vi "Generate Data.vi"() -> ()   [LabVIEW 2010]
doc: "이 VI는 LabVIEW Core II의 글로벌 데이터 프로젝트 연습문제에 대한 해답입니다.\n\n이 프로젝트를 실행하려면, 글로벌 데이터(Global Data) LV 프로젝트 파일을 열고, 데이터 생성(Generate Data) VI와 데이터 읽기(Read Data) VI를 열고, 실행하십시오. 데이터는 데이터 생성 VI에서 생성되며 데이터 읽기 VI에서 표시됩니다. 데이터 생성 VI와 데이터 읽기 VI는 하나의 정지 버튼을 공유합니다."
panel:
  out "데이터":dbl
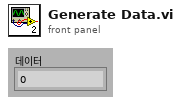
[diagram p1: front panel]
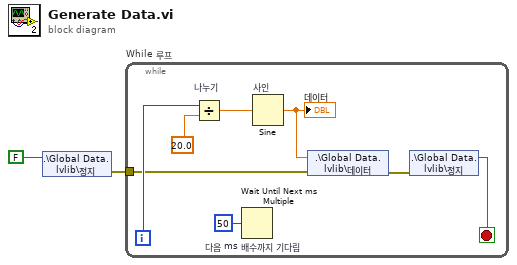
[diagram p0: block diagram]
diagram:
  n1 = shared-variable ".\\Global Data.lvlib\\정지"(FALSE ("Stop")) -> (error out=w1:errorcluster)  [unwired: 1 in]
  n2 = while "While 루프" {
    tunnel: w1 -> [w4]
    i -> [w10]
    stop <- w7 stop-if-true
    n3 = Divide "나누기"(x=w10, y=20.0) -> (x/y=w8:dbl)
    n4 = Wait Until Next ms Multiple "다음 ms 배수까지 기다림"(millisecond multiple=u32 50) -> ()  [unwired: 1 out]
    n5 = Sine "사인"(x=w8) -> (sin(x)=w6:dbl)
    "데이터" <- w6
    n6 = shared-variable ".\\Global Data.lvlib\\데이터"(w6, error in=w4) -> (error out=w3:errorcluster)
    n7 = shared-variable ".\\Global Data.lvlib\\정지"(error in=w3) -> (w7:bool)  [unwired: 1 out]
  }
